vi "autoDrive.vi"(3 "Rate":dbl=-4.0, 4 "Distance to Travel":dbl=-4.0) -> (0 "right speed":dbl, 1 "left speed":dbl, 2 "finished?":bool)   [LabVIEW 2013]
doc: "Will drive the robot at a specified speed for a specified distance. Pretty simple."
uses:
  typedefs/subStates.ctl
  <vilib>/addons/control/pid/pid.llb/PID Control Input Filter (DBL).vi
  <vilib>/addons/control/pid/pid.llb/PID (DBL).vi
  <vilib>/addons/control/pid/NI_PID_pid.lvlib
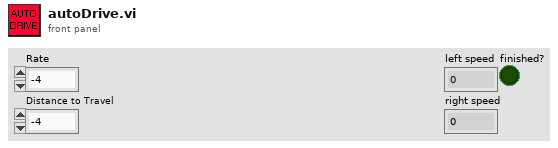
[diagram p1: front panel]
types:
  T1 = cluster{"proportional gain (Kc)":dbl, "integral time (Ti, min)":dbl, "derivative time (Td, min)":dbl}
  T2 = typedef "subStates.ctl" = enum16{"null", "wait", "driver control", "auto", "manual override", "hold position", "rotate", "pickup", "pass", "load", "goto shoot", "shoot high goal", "shoot low goal", "cancel arm", "cancel shooter", "end"}
  T3 = typedef "WPI_EncoderDevRef.ctl" = cluster{"DevStatus":errorcluster, "EncoderIndex":T4, "CounterIndex":T5, "DistancePerCount":dbl, "Decoding Type":T6}
  T4 = typedef "FPGA_EncoderIdx.ctl" = enum8{"Enc 0", "Enc 1", "Enc 2", "Enc 3", "Invalid"}
  T5 = typedef "FPGA_CounterCtrSystemIndex.ctl" = enum8{"Ctr 0", "Ctr 1", "Ctr 2", "Ctr 3", "Ctr 4", "Ctr 5", "Ctr 6", "Ctr 7", "Invalid"}
  T6 = typedef "WPI_EncoderType.ctl" = enum16{"1x", "2x", "4x"}
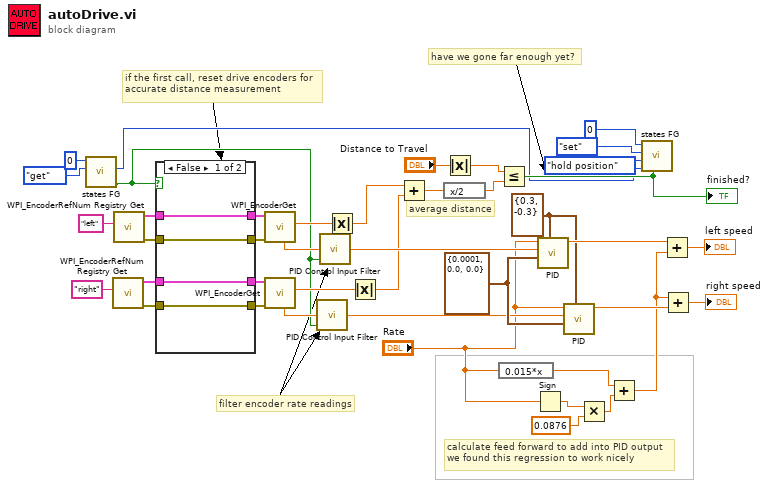
[diagram p0: block diagram]
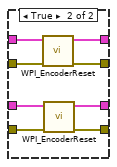
[diagram p2: hidden frame]
diagram:
  w40 = T1 {"proportional gain (Kc)"=0.0001, "integral time (Ti, min)"=0.0, "derivative time (Td, min)"=0.0} ("PID gains")
  w39 = cluster{"output high":dbl, "output low":dbl} {"output high"=0.3, "output low"=-0.3} ("output range")
  # "if the first call, reset drive encoders for accurate distance measurement"
  # "calculate feed forward to add into PID output\nwe found this regression to work nicely"
  # "have we gone far enough yet?"
  # "average distance"
  # "filter encoder rate readings"
  n1 = call "states FG.vi"("menu (get)"=enum16{"set", "get"}."get", "Loop ID"=0) -> ("first call?"=w11:bool, "state # out"=w1:i32)  [unwired: 6 in, 2 out]
  n2 = call <vilib>:"WPI_EncoderRefNum Registry Get.vi"("refnum name"="right") -> ("error out"=w22:errorcluster, "EncoderDevRef"=w23:T3)  [unwired: 9 in]
  n3 = call <vilib>:"WPI_EncoderRefNum Registry Get.vi"("refnum name"="left") -> ("error out"=w24:errorcluster, "EncoderDevRef"=w25:T3)  [unwired: 9 in]
  n4 = case shown="False" w11 {
    tunnel: w25 -> [w46 w52]
    tunnel: w24 -> [w45 w54]
    tunnel: w23 -> [w44 w49]
    tunnel: w22 -> [w43 w50]
    tunnel: [w45 w53] -> w21
    tunnel: [w46 w51] -> w20
    tunnel: [w44 w48] -> w19
    tunnel: [w43 w47] -> w18
    frame False {
    }
    frame True {
      n5 = call <vilib>:"WPI_EncoderReset.vi"("error in (no error)"=w54, "EncoderDevRef"=w52) -> ("error out"=w53:errorcluster, "EncoderDevRef"=w51:T3)  [unwired: 8 in]
      n6 = call <vilib>:"WPI_EncoderReset.vi"("error in (no error)"=w50, "EncoderDevRef"=w49) -> ("error out"=w47:errorcluster, "EncoderDevRef"=w48:T3)  [unwired: 8 in]
    }
  }
  n7 = call <vilib>:"WPI_EncoderGet.vi"("error in (no error)"=w21, "EncoderDevRef"=w20) -> ("Distance"=w17:dbl, "Rate"=w33:dbl)  [unwired: 4 in, 4 out]
  n8 = call <vilib>:"WPI_EncoderGet.vi"("error in (no error)"=w18, "EncoderDevRef"=w19) -> ("Distance"=w16:dbl, "Rate"=w32:dbl)  [unwired: 4 in, 4 out]
  n9 = call-poly <vilib>:"PID Control Input Filter.vi"("reinitialize? (F)"=w11, "input"=w32) -> ("output"=w12:dbl)  [unwired: 3 in]
  n10 = call-poly <vilib>:"PID Control Input Filter.vi"("reinitialize? (F)"=w11, "input"=w33) -> ("output"=w13:dbl)  [unwired: 3 in]
  n11 = Absolute Value(x=w17) -> (abs(x)=w10:dbl)
  n12 = Absolute Value(x=w16) -> (abs(x)=w9:dbl)
  n13 = Add(x=w10, y=w9) -> (x+y=w31:dbl)
  n14 = expression code="x/2"(w31) -> (w30:dbl)
  n15 = Absolute Value(x="Distance to Travel") -> (abs(x)=w2:dbl)
  n16 = Less Or Equal?(x=w2, y=w30) -> (x <= y?=w28:bool)
  "finished?" <- w28
  n17 = expression code="0.015*x"("Rate") -> (w5:dbl)
  n18 = Sign(1:"Rate") -> (0:w8:dbl)
  n19 = call-poly <vilib>:"PID.vi"("output range"=w39, "PID gains"=w40, "process variable"=w13, "setpoint"="Rate") -> ("output"=w41:dbl)  [unwired: 6 in, 1 out]
  n20 = call-poly <vilib>:"PID.vi"("output range"=w39, "PID gains"=w40, "process variable"=w12, "setpoint"="Rate") -> ("output"=w42:dbl)  [unwired: 6 in, 1 out]
  n21 = Multiply(x=w8, y=0.0876) -> (x*y=w6:dbl)
  n22 = Add(x=w5, y=w6) -> (x+y=w4:dbl)
  n23 = call "states FG.vi"("exit in"=w28, "state # in"=w1, "subState in"=subStates."hold position", "menu (get)"=enum16{"set", "get"}."set", "Loop ID"=0) -> ()  [unwired: 3 in, 4 out]
  n24 = Add(x=w41, y=w4) -> (x+y=→"left speed":dbl)
  n25 = Add(x=w4, y=w42) -> (x+y=→"right speed":dbl)
